vi "Read datatype.vi"(8 "error in (no error)":errorcluster, 11 "PointerInt32Datatype in":refnum<class "PointerInt32Datatype.lvclass">) -> (0 "error out":errorcluster, 2 "datatype":string="int32*", 3 "PointerInt32Datatype out":refnum<class "PointerInt32Datatype.lvclass">)   [LabVIEW 2014, in "PointerInt32Datatype.lvclass"]
uses:
  PointerInt32Datatype.lvclass
  PointerInt32Datatype.lvclass/PointerInt32Datatype.ctl
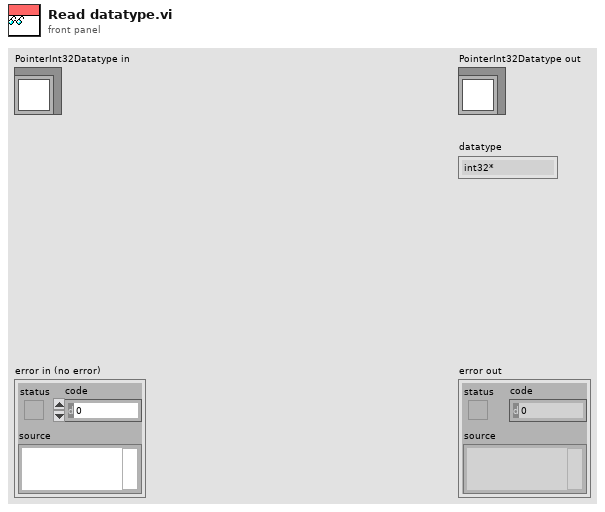
[diagram p1: front panel]
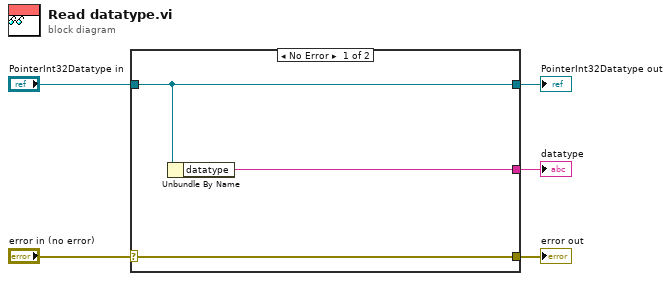
[diagram p0: block diagram]
diagram:
  n1 = case shown="No Error" "error in (no error)" {
    selector: "error in (no error)" -> [w8 w9]
    tunnel: [w8 w9] -> w4
    tunnel: [w7 w10] -> w2
    tunnel: "PointerInt32Datatype in" -> [w7 w10]
    tunnel: [w6 _] -> w1
    frame No Error {
      n2 = Unbundle By Name(w7) -> ("datatype"=w6:string)
    }
    frame Error {
    }
  }
  "error out" <- w4
  "PointerInt32Datatype out" <- w2
  "datatype" <- w1
